vi "Link Children.vi"(8 "error in (no error)":errorcluster, 11 "xml structure":T1) -> (0 "error out":errorcluster, 3 "xml structure out":T1)   [LabVIEW 2011]
uses:
  XML Structure - Cluster.ctl
  XML Tag Type - Enum.ctl
  <userlib>/_OpenG.lib/array/array.llb/Conditional Auto-Indexing Tunnel (I32)__ogtk.vi
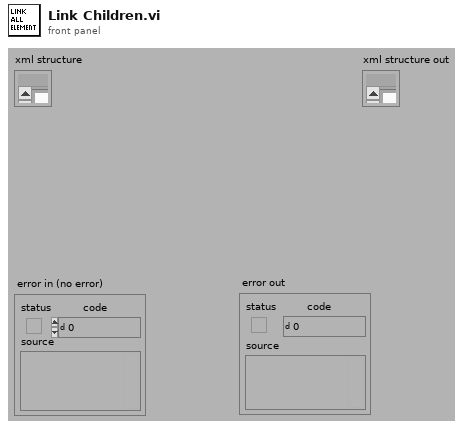
[diagram p1: front panel]
types:
  T1 = typedef "XML Structure - Cluster.ctl" = cluster{"tags":string[], "tag names":string[], "tag type":T2[], "offset":i32[], "close tag index":i32[], "xml":string, "Children":cluster{"children":i32[]}[], "parent index":i32[]}
  T2 = typedef "XML Tag Type - Enum.ctl" = enum16{"start tag", "empty tag", "end tag"}
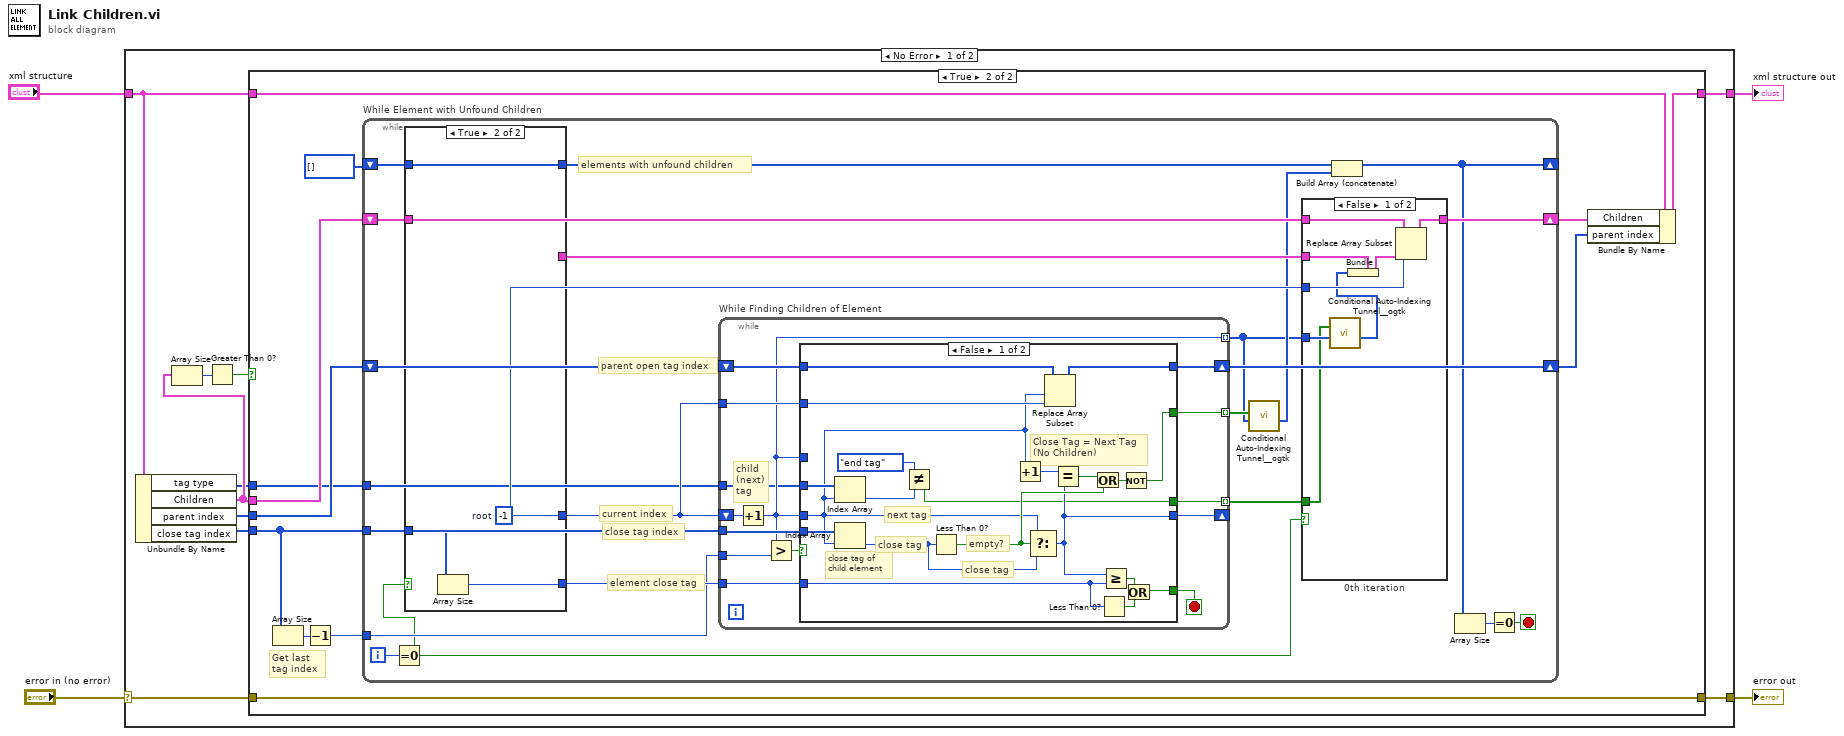
[diagram p0: block diagram]
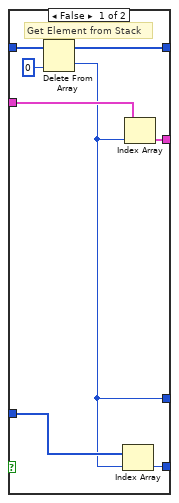
[diagram p3: hidden frame]
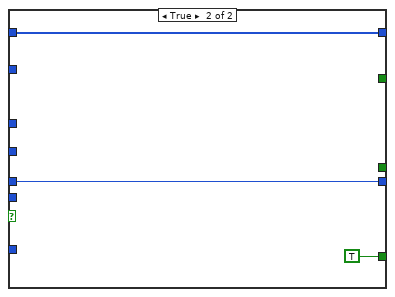
[diagram p5: hidden frame]
diagram:
  n1 = case shown="No Error" "error in (no error)" {
    selector: "error in (no error)" -> [w8 w108]
    tunnel: "xml structure" -> [w13 w109]
    tunnel: [w11 w109] -> w3
    tunnel: [w9 w108] -> w1
    frame No Error {
      n2 = Unbundle By Name(w13) -> ("tag type"=w5:T2[], "Children"=w10:cluster{"children":i32[]}[], "parent index"=w12:i32[], "close tag index"=w14:i32[])
      n3 = Array Size(array=w10) -> (size(s)=w6:i32)
      n4 = Greater Than 0?(x=w6) -> (x > 0?=w7:bool)
      n5 = case shown="True" w7 {
        tunnel: w14 -> [_ w21]
        tunnel: w13 -> [w16 w28]
        tunnel: w12 -> [_ w25]
        tunnel: [w16 w24] -> w11
        tunnel: w10 -> [_ w23]
        tunnel: [w15 w22] -> w9
        tunnel: w8 -> [w15 w22]
        tunnel: w5 -> [_ w18]
        frame False {
        }
        frame True {
          # "Get last tag index"
          n6 = Array Size(array=w21) -> (size(s)=w20:i32)
          n7 = Decrement(x=w20) -> (x-1=w19:i32)
          n8 = while "While Element with Unfound Children" {
            shift-right: [w41] -> w26
            shift-left: w25 -> [w45]
            shift-right: [w35] -> _
            shift-left: i32[] [] -> [w49]
            shift-right: [w42] -> w27
            shift-left: w23 -> [w43]
            tunnel: w21 -> [w44]
            tunnel: w19 -> [w33]
            tunnel: w18 -> [w30]
            i -> [w36]
            stop <- w46 stop-if-true
            # "current index"
            # "element close tag"
            # "elements with unfound children"
            # "parent open tag index"
            # "close tag index"
            n9 = Equal To 0?(x=w36) -> (x = 0?=w29:bool)
            n10 = case shown="True" w29 {
              tunnel: w49 -> [w57 w61]
              tunnel: [w56 w61] -> w48
              tunnel: w44 -> [w54 w59]
              tunnel: w43 -> [w53 _]
              tunnel: [w52 _] -> w40
              tunnel: [w51 w60] -> w39
              tunnel: [w50 w58] -> w37
              frame False {
                # "Get Element from Stack"
                n11 = Delete From Array(array=w57, index=0) -> (deleted portion=w51:i32, array with subset deleted=w56:i32[])  [unwired: 1 in]
                n12 = Index Array(array=w54, index=w51) -> (element=w50:i32)
                n13 = Index Array(array=w53, index=w51) -> (element=w52:cluster{"children":i32[]})
              }
              frame True {
                w60 = -1  # root
                n14 = Array Size(array=w59) -> (size(s)=w58:i32)
              }
            }
            n15 = while "While Finding Children of Element" {
              shift-right: [w77] -> _
              shift-left: w39 -> [w84]
              tunnel: w37 -> [w78]
              tunnel: [w74] -> w32 mode=indexing
              tunnel: [w79] -> w38 mode=indexing
              shift-right: [w82] -> w41
              shift-left: w45 -> [w83]
              tunnel: w44 -> [w81]
              tunnel: w39 -> [w80]
              tunnel: w33 -> [w76]
              tunnel: [w72] -> w31 mode=indexing
              tunnel: w30 -> [w71]
              stop <- w73 stop-if-true
              # "child (next) tag"
              n16 = Increment(x=w84) -> (x+1=w74:i32)
              n17 = Greater?(x=w74, y=w76) -> (0:w75:bool)
              n18 = case shown="False" w75 {
                tunnel: w83 -> [w103 w107]
                tunnel: [w102 w107] -> w82
                tunnel: w81 -> [w101 _]
                tunnel: w80 -> [w99 _]
                tunnel: [w97 _] -> w79
                tunnel: w78 -> [w85 _]
                tunnel: [w95 w106] -> w77
                tunnel: [w94 TRUE] -> w73
                tunnel: w74 -> [w89 w106]
                tunnel: w74 -> [_ _]
                tunnel: [w86 _] -> w72
                tunnel: w71 -> [w90 _]
                frame False {
                  # "Close Tag = Next Tag\n(No Children)"
                  # "close tag"
                  # "next tag"
                  # "empty?"
                  # "close tag of child element"
                  # "close tag"
                  n19 = Index Array(array=w90, index=w89) -> (element=w88:T2)
                  n20 = Index Array(array=w101, index=w89) -> (element=w100:i32)
                  n21 = Not Equal?(x=XML_Tag_Type_-_Enum."end tag", y=w88) -> (x != y?=w86:bool)
                  n22 = Less Than 0?(x=w100) -> (x < 0?=w96:bool)
                  n23 = Increment(x=w89) -> (x+1=w104:i32)
                  n24 = Select(t=w89, s=w96, f=w100) -> (s? t:f=w95:i32)
                  n25 = Replace Array Subset(array=w103, new element=w99, index=w89) -> (w102:i32[])
                  n26 = Equal?(x=w104, y=w95) -> (x = y?=w91:bool)
                  n27 = Or(x=w91, y=w96) -> (x .or. y?=w98:bool)
                  n28 = Less Than 0?(x=w85) -> (x < 0?=w93:bool)
                  n29 = Greater Or Equal?(x=w95, y=w85) -> (x >= y?=w92:bool)
                  n30 = Not(x=w98) -> (.not. x?=w97:bool)
                  n31 = Or(x=w92, y=w93) -> (x .or. y?=w94:bool)
                }
                frame True {
                }
              }
            }
            n32 = call-poly <userlib>:"Conditional Auto-Indexing Tunnel__ogtk.vi"("Array in"=w32, "Elements to keep"=w38) -> ("Filtered Array out"=w34:i32[])  [unwired: 5 in]
            n33 = case "0th iteration" shown="False" w29 {
              tunnel: w43 -> [w69 w70]
              tunnel: [w67 w70] -> w42
              tunnel: w40 -> [w66 _]
              tunnel: w39 -> [w65 _]
              tunnel: w32 -> [w64 _]
              tunnel: w31 -> [w62 _]
              frame False {
                n34 = call-poly <userlib>:"Conditional Auto-Indexing Tunnel__ogtk.vi"("Array in"=w64, "Elements to keep"=w62) -> ("Filtered Array out"=w63:i32[])  [unwired: 5 in]
                n35 = Bundle(cluster=w66, "children"=w63) -> (w68:cluster{"children":i32[]})
                n36 = Replace Array Subset(array=w69, new element=w68, index=w65) -> (w67:cluster{"children":i32[]}[])
              }
              frame True {
              }
            }
            n37 = Build Array (concatenate)(w48, w34) -> (w35:i32[])
            n38 = Array Size(array=w35) -> (size(s)=w47:i32)
            n39 = Equal To 0?(x=w47) -> (x = 0?=w46:bool)
          }
          n40 = Bundle By Name(cluster=w28, "Children"=w27, "parent index"=w26) -> (w24:T1)
        }
      }
    }
    frame Error {
    }
  }
  "xml structure out" <- w3
  "error out" <- w1
